vi "GetRTTemplateFile.vi"(8 "error in (no error)":errorcluster, 11 "absolute custom device xml file":path) -> (0 "error out":errorcluster, 3 "connector pane template":T1)   [LabVIEW 2015, in "VeriStandTestCase.lvclass"]
uses:
  VeriStandTestCase.lvclass
  ConnectorPaneTemplate.ctl
  <vilib>/xml/Load XML File.vi
  <vilib>/xml/Close Reference(Node).vi
  <userlib>/_OpenG.lib/file/file.llb/Build Path - Traditional - path__ogtk.vi
  <vilib>/xml/NI_XML.lvlib
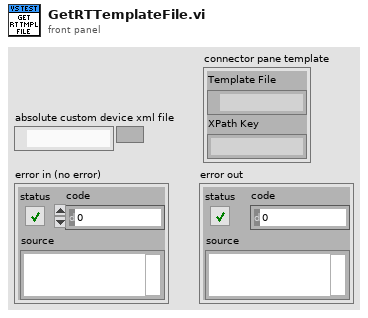
[diagram p1: front panel]
types:
  T1 = typedef "VeriStandTestCase.lvclass/ConnectorPaneTemplate.ctl" = cluster{"Template File":path, "XPath Key":string}
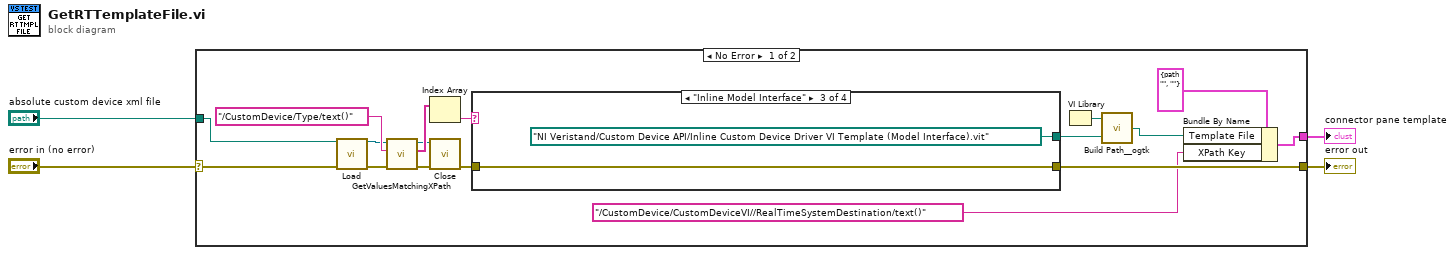
[diagram p0: block diagram]
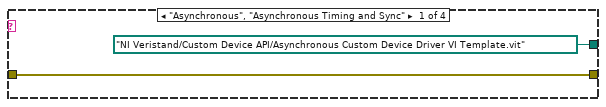
[diagram p2: hidden frame]
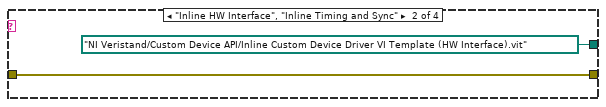
[diagram p3: hidden frame]
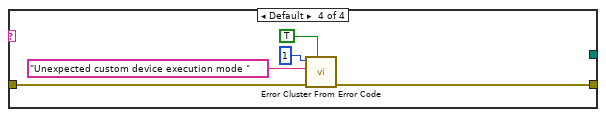
[diagram p4: hidden frame]
diagram:
  n1 = case shown="No Error" "error in (no error)" {
    selector: "error in (no error)" -> [w21 w33]
    tunnel: "absolute custom device xml file" -> [w18 _]
    tunnel: [w11 w33] -> w2
    tunnel: [w9 _] -> w1
    frame No Error {
      n2 = call-poly <vilib>:"Load.vi"("path to XML document"=w18, "error in (no error)"=w21) -> ("DOM document out"=w14:refnum<k20>, "error out"=w16:errorcluster)  [unwired: 11 in, 1 out]
      n3 = call "GetValuesMatchingXPath.vi"("error in (no error)"=w16, "XPath"="/CustomDevice/Type/text()", "XML refnum in"=w14) -> ("error out"=w17:errorcluster, "Values"=w15:string[], "XML refnum out"=w13:refnum<k20>)  [unwired: 6 in]
      n4 = Index Array(array=w15) -> (element=w20:string)  [unwired: 1 in]
      n5 = call-poly <vilib>:"Close.vi"("error in (no error)"=w17, "node"=w13) -> ("error out"=w12:errorcluster)  [unwired: 7 in]
      n6 = case shown="\"Inline Model Interface\"" w20 {
        tunnel: [path "NI Veristand/Custom Device API/Asynchronous Custom Device Driver VI Template.vit" ("Folder Path") path "NI Veristand/Custom Device API/Inline Custom Device Driver VI Template (HW Interface).vit" ("Folder Path") path "NI Veristand/Custom Device API/Inline Custom Device Driver VI Template (Model Interface).vit" ("Folder Path") _] -> w6
        tunnel: w12 -> [w22 w24 w26 w32]
        tunnel: [w22 w24 w26 w31] -> w11
        frame "Asynchronous", "Asynchronous Timing and Sync" {
        }
        frame "Inline HW Interface", "Inline Timing and Sync" {
        }
        frame "Inline Model Interface" {
        }
        frame Default {
          n7 = call <vilib>:"Error Cluster From Error Code.vi"("show call chain? (False)"=TRUE, "error in (no error)"=w32, "error message (\"\")"="Unexpected custom device execution mode " ("error message (\"\")"), "error code (0)"=1) -> ("error out"=w31:errorcluster)  [unwired: 5 in]
        }
      }
      n8 = VI Library() -> (path=w7:path)
      n9 = call-poly <userlib>:"Build Path__ogtk.vi"("name or relative path"=w6, "base path"=w7) -> ("appended path"=w5:path)
      n10 = Bundle By Name(cluster=T1 {"Template File"=path "", "XPath Key"=""} ("connector pane template 2"), "Template File"=w5, "XPath Key"="/CustomDevice/CustomDeviceVI//RealTimeSystemDestination/text()") -> (w9:T1)
    }
    frame Error {
    }
  }
  "error out" <- w2
  "connector pane template" <- w1
